vi "Single Read.vi"(9 "Tree":string(tree), 10 "Tree Ref":refnum<vi>) -> (2 "Cell String":string)   [LabVIEW 2020, in "_Shared.lvlib" / "Tree.lvlib"]
uses:
  Tree.lvlib
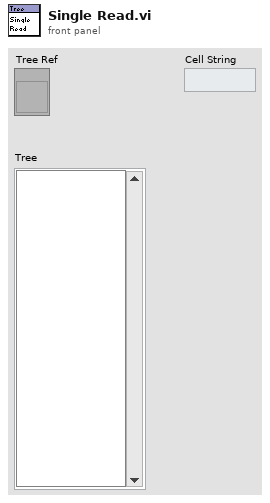
[diagram p1: front panel]
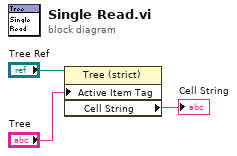
[diagram p0: block diagram]
diagram:
  n1 = property class="Tree (strict)"(reference="Tree Ref", "Active Item Tag"="Tree") -> ("Cell String"=→"Cell String":string)  [unwired: 1 in, 2 out]
